vi "Repeated Start.vi"(8 "error in (no error)":errorcluster, 11 "Low Speed in":refnum<class "Low Speed.lvclass">) -> (0 "error out":errorcluster, 3 "Low Speed out":refnum<class "Low Speed.lvclass">)   [LabVIEW 2020, in "Low Speed.lvclass"]
uses:
  Low Speed.lvclass
  C:/Users/kaiser.asan/OneDrive - SolitonTechnologies/LabVIEW/29.SDLC - I2C Driver/I2C Module/I2C Controller Module/Class/Transmission Mode/Parent/TX Speed.lvclass
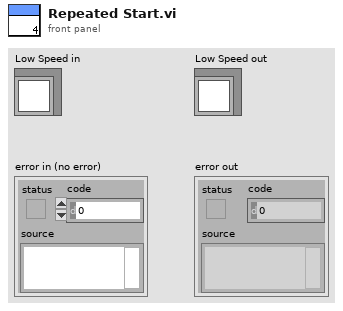
[diagram p1: front panel]
types:
  T1 = typedef "I2C Controller Lib.lvlib/Timing Parameters Cluster.ctl" = cluster{"f_SCL(KHz)":u32, "t_HIGH (ns)":u32, "t_LOW (ns)":u32, "t_SU;STA (ns)":u32, "t_HD;STA (ns)":u32, "t_SU;DAT (ns)":u32, "t_HD;DAT (ns)":u32, "t_SU;STO (ns)":u32, "t_BUF (ns)":u32}
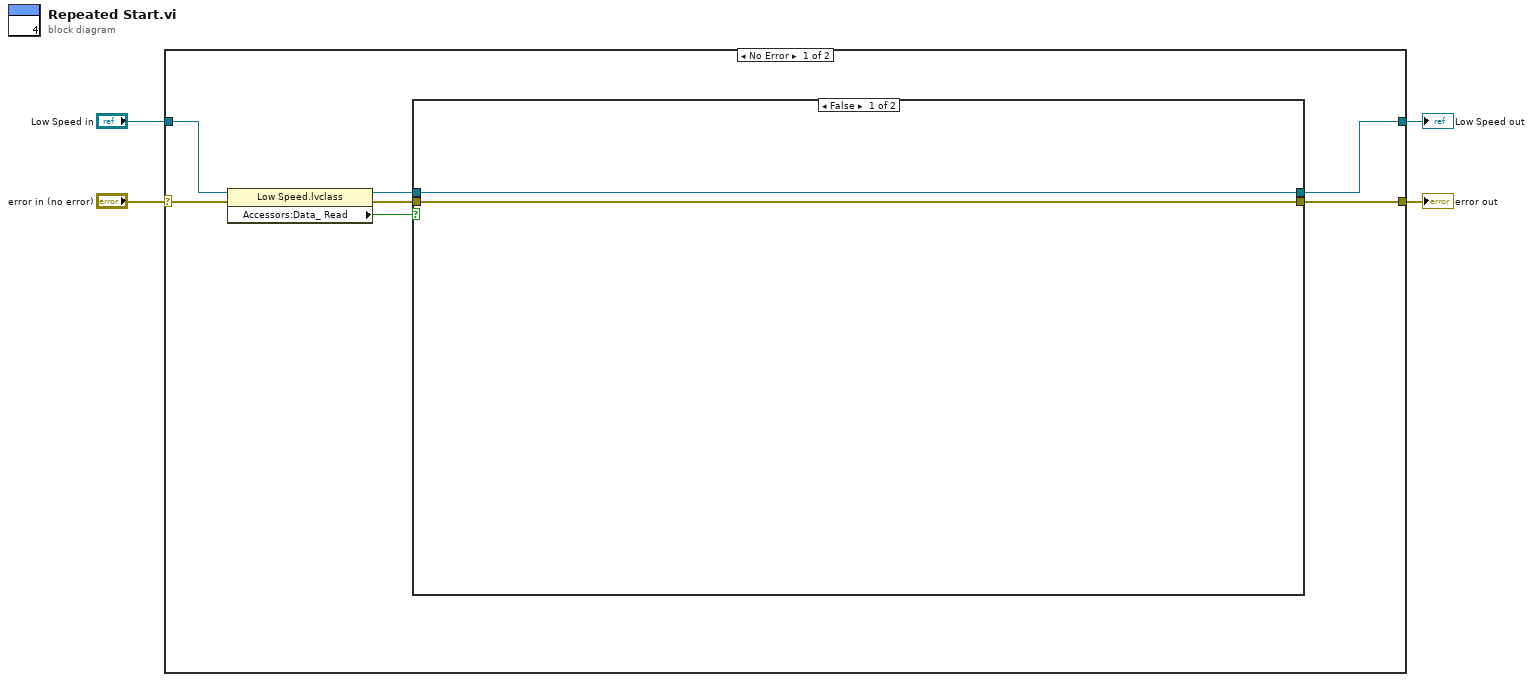
[diagram p0: block diagram]
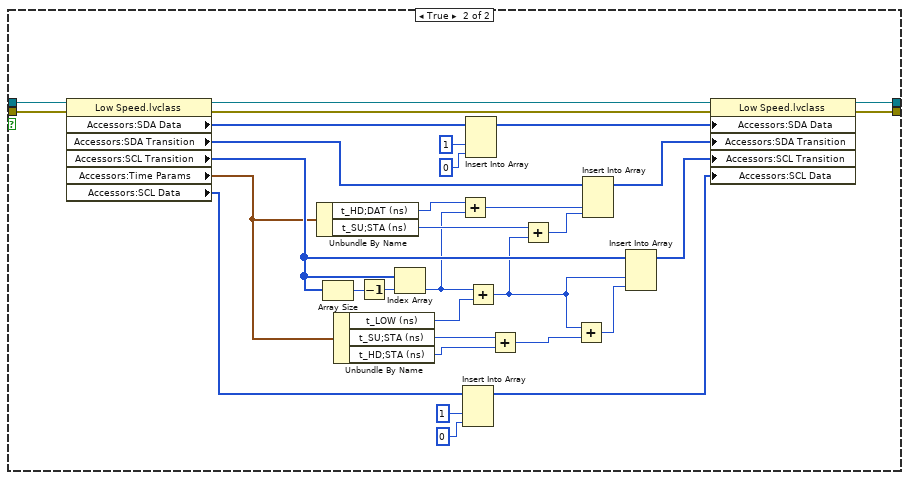
[diagram p2: hidden frame]
diagram:
  n1 = case shown="No Error" "error in (no error)" {
    selector: "error in (no error)" -> [w11 w46]
    tunnel: [w10 w46] -> w4
    tunnel: [w9 w47] -> w2
    tunnel: "Low Speed in" -> [w7 w47]
    frame No Error {
      n2 = property class="Low Speed.lvclass"(reference=w7, error in=w11) -> (reference out=w6:refnum<class "Low Speed.lvclass">, error out=w8:errorcluster, "Accessors:Data_ Read"=w5:bool)
      n3 = case shown="False" w5 {
        tunnel: w8 -> [w12 w45]
        tunnel: w6 -> [w13 w43]
        tunnel: [w12 w42] -> w10
        tunnel: [w13 w40] -> w9
        frame False {
        }
        frame True {
          n4 = property class="Low Speed.lvclass"(reference=w43, error in=w45) -> (reference out=w41:refnum<class "Low Speed.lvclass">, error out=w44:errorcluster, "Accessors:SDA Data"=w39:u8[], "Accessors:SDA Transition"=w35:u32[], "Accessors:SCL Transition"=w29:u32[], "Accessors:Time Params"=w28:T1, "Accessors:SCL Data"=w22:u8[])
          n5 = Unbundle By Name(w28) -> ("t_HD;DAT (ns)"=w18:u32, "t_SU;STA (ns)"=w16:u32)
          n6 = Array Size(array=w29) -> (size(s)=w33:i32)
          n7 = Unbundle By Name(w28) -> ("t_LOW (ns)"=w31:u32, "t_SU;STA (ns)"=w26:u32, "t_HD;STA (ns)"=w24:u32)
          n8 = Decrement(x=w33) -> (x-1=w32:i32)
          n9 = Index Array(array=w29, index=w32) -> (element=w14:u32)
          n10 = Add(x=w18, y=w14) -> (x+y=w17:u32)
          n11 = Insert Into Array(array=w22, new element #1=u8 1 ("new element/subarray"), new element #2=u8 0 ("new element/subarray")) -> (w21:u8[])  [unwired: 1 in]
          n12 = Insert Into Array(array=w39, new element #1=u8 1 ("new element/subarray"), new element #2=u8 0 ("new element/subarray")) -> (w38:u8[])  [unwired: 1 in]
          n13 = Add(x=w14, y=w31) -> (x+y=w15:u32)
          n14 = Add(x=w26, y=w24) -> (x+y=w25:u32)
          n15 = Add(x=w16, y=w15) -> (x+y=w19:u32)
          n16 = Add(x=w15, y=w25) -> (x+y=w30:u32)
          n17 = Insert Into Array(array=w35, new element #1=w17, new element #2=w19) -> (w34:u32[])  [unwired: 1 in]
          n18 = Insert Into Array(array=w29, new element #1=w15, new element #2=w30) -> (w27:u32[])  [unwired: 1 in]
          n19 = property class="Low Speed.lvclass"(reference=w41, error in=w44, "Accessors:SDA Data"=w38, "Accessors:SDA Transition"=w34, "Accessors:SCL Transition"=w27, "Accessors:SCL Data"=w21) -> (reference out=w40:refnum<class "Low Speed.lvclass">, error out=w42:errorcluster)
        }
      }
    }
    frame Error {
    }
  }
  "error out" <- w4
  "Low Speed out" <- w2
